vi "DVR LV2.vi"(0 "Data Value Reference":refnum<data-value>, 11 "error in (no error)":errorcluster, 13 "Operation":T1) -> (4 "Data Value Reference Out":refnum<data-value>, 15 "error out":errorcluster)   [LabVIEW 2023]
doc: "This Vi acts as a LV2 global for storing the data value reference."
uses:
  Controls/StoreRef.ctl
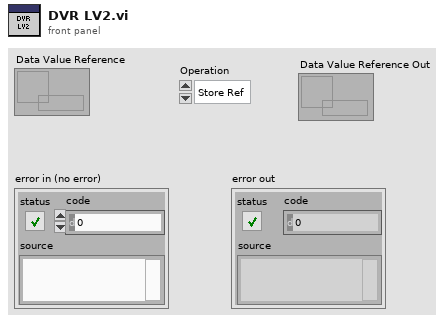
[diagram p1: front panel]
types:
  T1 = typedef "StoreRef.ctl" = enum16{"Store Ref", "Get Ref"}
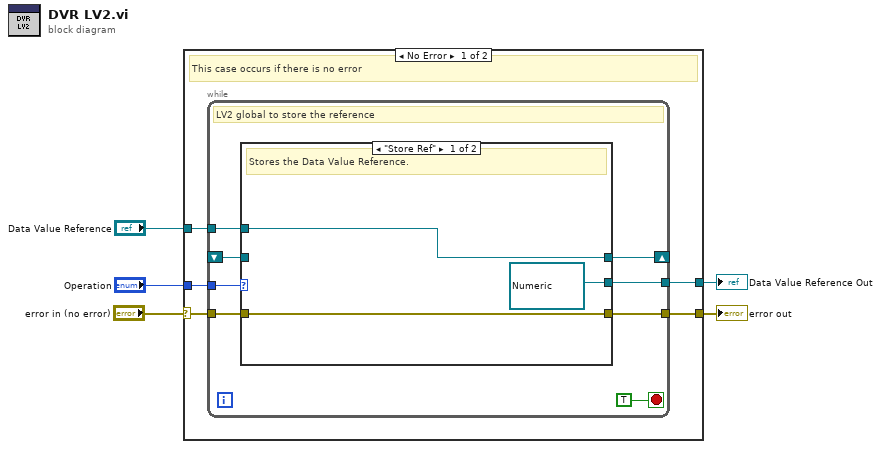
[diagram p0: block diagram]
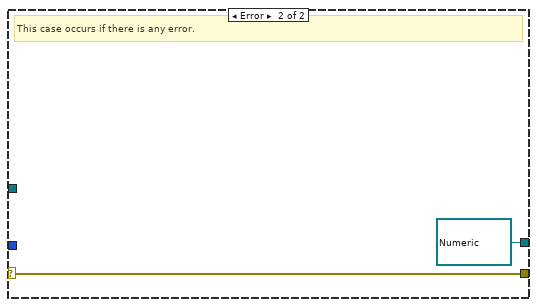
[diagram p3: hidden frame]
diagram:
  n1 = case shown="No Error" "error in (no error)" {
    selector: "error in (no error)" -> [w10 w25]
    tunnel: "Operation" -> [w9 _]
    tunnel: [w8 w25] -> w3
    tunnel: "Data Value Reference" -> [w7 _]
    tunnel: [w6 refnum<data-value> refnum ("Data Value Reference")] -> w1
    frame No Error {
      # "This case occurs if there is no error"
      n2 = while {
        tunnel: w10 -> [w18]
        tunnel: w9 -> [w17]
        tunnel: [w16] -> w8
        shift-right: [w14] -> _
        shift-left: _ -> [w15]
        tunnel: w7 -> [w13]
        tunnel: [w12] -> w6
        stop <- TRUE stop-if-true
        # "LV2 global to store the reference"
        n3 = case shown="\"Store Ref\"" w17 {
          tunnel: [w21 w23] -> w16
          tunnel: w18 -> [w21 w23]
          tunnel: w15 -> [_ w22]
          tunnel: [w20 w22] -> w14
          tunnel: w13 -> [w20 _]
          tunnel: [refnum<data-value> refnum ("data value reference") w22] -> w12
          frame "Store Ref" {
            # "Stores the Data Value Reference."
          }
          frame "Get Ref" {
            # "Gives the stored Data Value Reference out to indicator."
          }
        }
      }
    }
    frame Error {
      # "This case occurs if there is any error."
    }
  }
  "error out" <- w3
  "Data Value Reference Out" <- w1
